vi "monochromatorCommandGetShutter.vi"(8 "error in":errorcluster, 11 "monochromator":refnum<k24>) -> (0 "error out":errorcluster, 1 "shutterTxt":string, 2 "shutter":bool, 3 "monochromator":refnum<k24>)   [LabVIEW 2009]
doc: "Get shutter status\nFALSE = Shutter is CLOSED\nTRUE = Shutter is OPEN"
uses:
  C:/Users/anderson.chen/Desktop/Software Development/Cornerstone Series API (LV9)/Cornerstone DLL/Cornerstone.dll
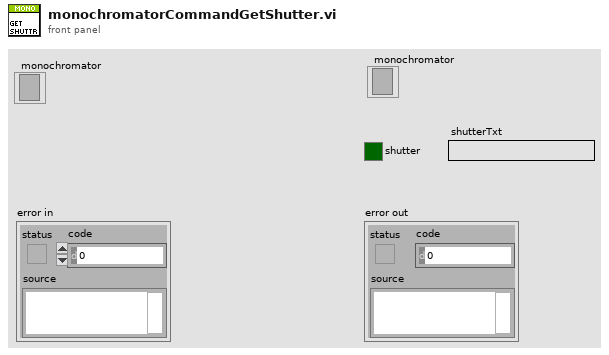
[diagram p1: front panel]
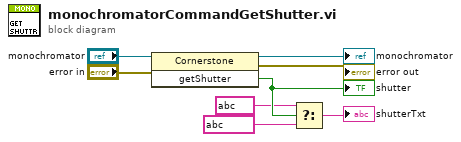
[diagram p0: block diagram]
diagram:
  n1 = invoke class="Cornerstone" method="getShutter"(reference="monochromator", error in="error in") -> (reference out=→"monochromator":refnum<k24>, error out=→"error out":errorcluster, "getShutter"=w4:bool)  [unwired: 1 in]
  "shutter" <- w4
  n2 = Select(t=string ?, s=w4, f=string ?) -> (s? t:f=→"shutterTxt":string)
